vi "SeCrTS-DD DI Search Channel dis.vi"(11 "DI Data":digitalwaveform[](array[waveform])) -> (3 "Array 2":bool[](array[boolean]))   [LabVIEW 2022 SP3]
uses:
  <vilib>/Waveform/DTblOps.llb/DTbl Digital to Boolean Array.vi
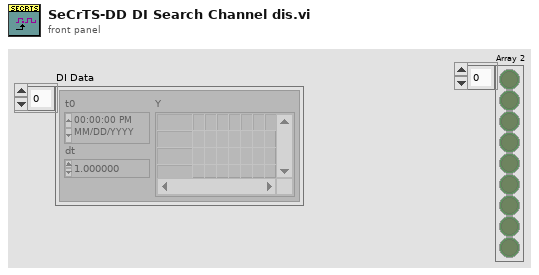
[diagram p1: front panel]
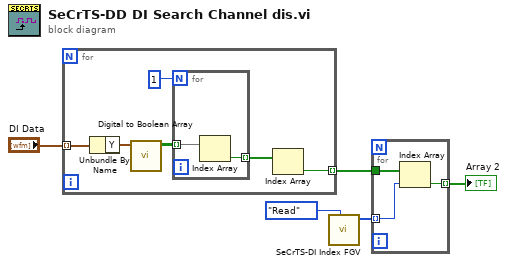
[diagram p0: block diagram]
diagram:
  n1 = for {
    tunnel: "DI Data" -> [w8] mode=indexing
    tunnel: [w6] -> w3 mode=indexing
    n2 = Unbundle By Name(w8) -> ("Y"=w9:digitaldata)
    n3 = call-poly <vilib>:"Digital to Boolean Array.vi"("digital data"=w9) -> ("boolean array"=w10:bool[][])  [unwired: 9 in, 1 out]
    n4 = for {
      N: 1 -> [_]
      tunnel: w10 -> [w13] mode=indexing
      tunnel: [w12] -> w7 mode=indexing
      n5 = Index Array(array=w13) -> (element=w12:bool)  [unwired: 1 in]
    }
    n6 = Index Array(array=w7) -> (element=w6:bool)  [unwired: 1 in]
  }
  n7 = call "SeCrTS-DI Index FGV .vi"("Action"=enum16{"Write", "Read", "Init"}."Read") -> ("Ai Index Element R"=w2:i32[])  [unwired: 10 in]
  n8 = for {
    tunnel: w3 -> [w16]
    tunnel: w2 -> [w15] mode=indexing
    tunnel: [w14] -> w1 mode=indexing
    n9 = Index Array(array=w16, index=w15) -> (element=w14:bool)
  }
  "Array 2" <- w1
